vi "Log Info.vi"(7 "Source":string, 8 "error in (no error)":errorcluster, 10 "Message":string, 11 "Logging In":refnum<class "Logging.lvclass">) -> (0 "error out":errorcluster, 3 "Logging Out":refnum<class "Logging.lvclass">)   [LabVIEW 2021, in "Logging.lvclass"]
doc: "Enter an info-level message into the system log.\nInfo implies a confirmation that things are working as expected."
uses:
  Logging.lvclass
  Protected/Level.ctl
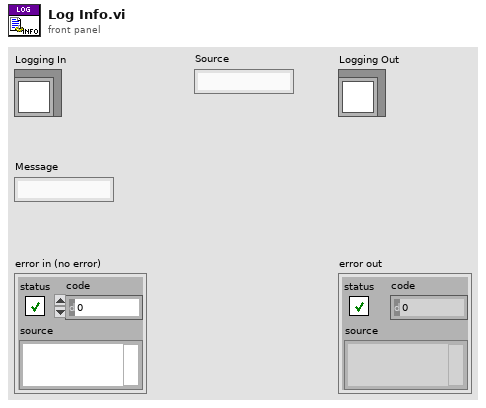
[diagram p1: front panel]
types:
  T1 = typedef "Logging.lvclass/Level.ctl" = enum16{"DEBUG", "INFO", "WARNING", "ERROR", "CRITICAL"}
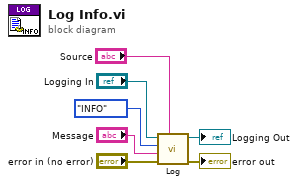
[diagram p0: block diagram]
diagram:
  n1 = call-dynamic "Log.vi"("Source"="Source", "error in (no error)"="error in (no error)", "Message"="Message", "Level"=Level."INFO", "Logging In"="Logging In") -> ("error out"=→"error out":errorcluster, "Logging Out"=→"Logging Out":refnum<class "Logging.lvclass">)  [unwired: 5 in]
